vi "C4Dev_stopAcquisition.vi"(0 "c4dev in":refnum<k24>, 11 "error in (no error)":errorcluster) -> (4 "c4dev out":refnum<k24>, 15 "error out":errorcluster)   [LabVIEW 2015, in "libC4HdlLV.lvlib"]
uses:
  libC4HdlLV.lvlib
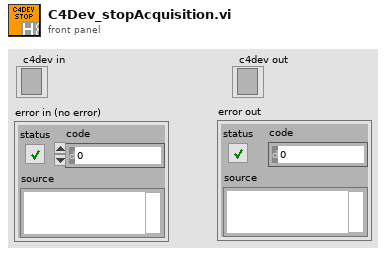
[diagram p1: front panel]
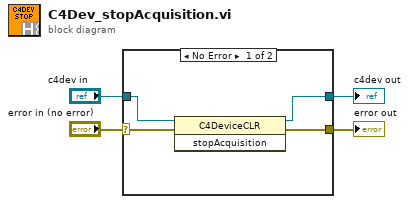
[diagram p0: block diagram]
diagram:
  n1 = case shown="No Error" "error in (no error)" {
    selector: "error in (no error)" -> [w5 w10]
    tunnel: "c4dev in" -> [w8 w9]
    tunnel: [w7 w9] -> w1
    tunnel: [w6 w10] -> w4
    frame No Error {
      n2 = invoke class="C4DeviceCLR" method="stopAcquisition"(reference=w8, error in=w5) -> (reference out=w7:refnum<k24>, error out=w6:errorcluster)  [unwired: 1 in, 1 out]
    }
    frame Error {
    }
  }
  "error out" <- w4
  "c4dev out" <- w1
